vi "Scales Page.vi"() -> ()   [LabVIEW 2020, in "2D Plot.lvclass"]
uses:
  <vilib>/Math Plots/2D Math Plots/2D Plot/2D Plot/2D Plot.lvclass
  <vilib>/Math Plots/2D Math Plots/2D Plot/2D Plot/Typedef/Scale Array.ctl
  <vilib>/Math Plots/2D Math Plots/2D Plot/2D Plot/Typedef/Scale Cluster.ctl
  <vilib>/Utility/miscctls.llb/LVOffsetAndMultiplierTypeDef.ctl
  <vilib>/Math Plots/2D Math Plots/2D Plot/Action String/2DMathPlot Ctrl Act Queue.ctl
  <vilib>/Math Plots/2D Math Plots/2D Plot/Action String/2DMathPlot Ctrl Act Cluster.ctl
  <vilib>/Math Plots/2D Math Plots/2D Plot/Action String/2DMathPlot State Class.ctl
  <vilib>/Math Plots/2D Math Plots/2D Plot/2D Plot/Typedef/Dialog State.ctl
  <vilib>/Math Plots/2D Math Plots/2D Plot/2D Plot/Typedef/Temp Graph State.ctl
  <vilib>/Math Plots/2D Math Plots/2D Plot/2D Plot/Typedef/Temp Graph Property Action.ctl
panel:
  in  "Axis":string[](array[string])=["(X-Axis)", "(Y-Axis)"]
  in  "R Axis":string[](array[string])=["(R-Axis)"]
  in  "Event Registration":refnum<event-registration>
  in  "Control Ref Queue":T1
  out "Scale Array Out":T2
  in  "Scale Array In":T2
  in  "Current Scale":u16(ring) caption="Axes" items=["Time(X-Axis)", "Amplitude(Y-Axis)"]
  in  "Multiplier":dbl
  in  "Offset":dbl
  in  "Scale Style":u16(ring) caption="Scale Style and Colors"
  in  "Grid Style":u16(ring) caption="Grid Style and Colors"
  in  "Show Scale Label":bool caption="Show scale label"
  in  "Maximum":dbl=10.0
  in  "Minimum":dbl
  in  "Minor Grid":u32(colorbox)=13056 caption="Minor grid"
  in  "Major Grid":u32(colorbox)=26112 caption="Major grid"
  in  "Marker Text":u32(colorbox) caption="Marker text"
  in  "Minor Tick":u32(colorbox) caption="Minor tick"
  in  "Major Tick":u32(colorbox) caption="Major tick"
  in  "Autoscale":bool
  in  "Log":bool
  in  "Show Scale":bool caption="Show scale"
  in  "Inverted":bool
  in  "Name":string
  # "Scaling Factors"
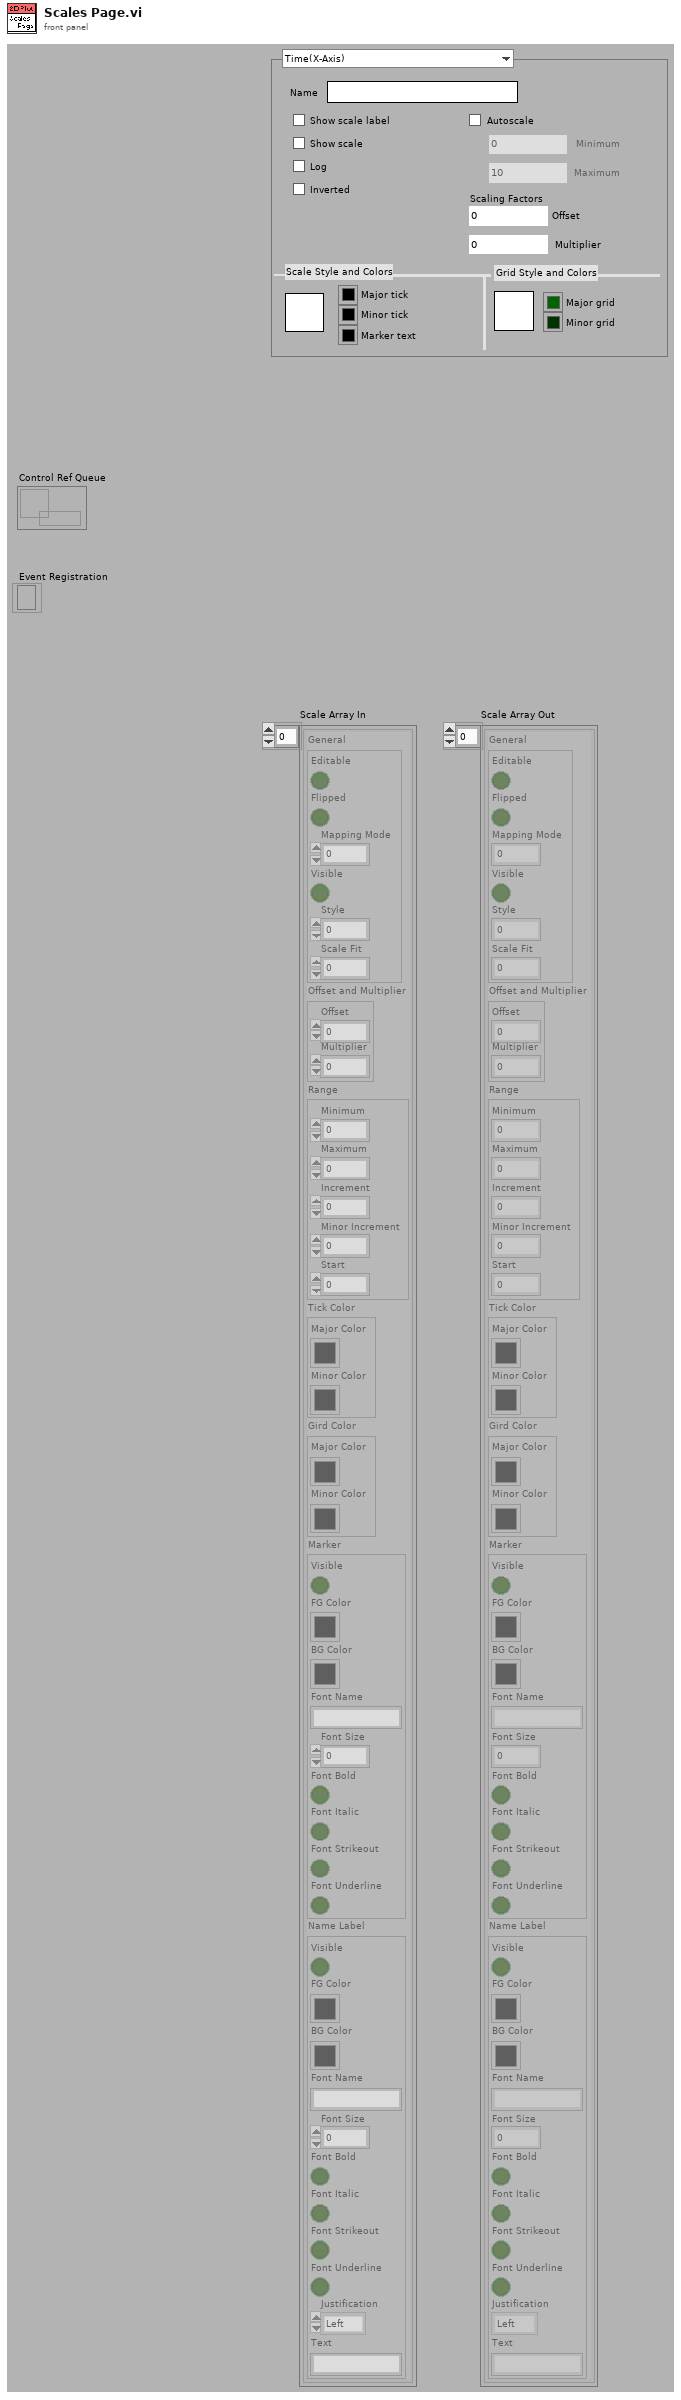
[diagram p1: front panel]
types:
  T1 = typedef "2DMathPlot Ctrl Act Queue.ctl" = refnum<queue>
  T2 = typedef "2D Plot.lvclass/Scale Array.ctl" = T3[]
  T3 = typedef "2D Plot.lvclass/Scale Cluster.ctl" = cluster{"General":cluster{"Editable":bool, "Flipped":bool, "Mapping Mode":u8, "Visible":bool, "Style":u8, "Scale Fit":u8}, "Offset and Multiplier":T4, "Range":cluster{"Minimum":dbl, "Maximum":dbl, "Increment":dbl, "Minor Increment":dbl, "Start":dbl}, "Tick Color":cluster{"Major Color":u32, "Minor Color":u32}, "Gird Color":cluster{"Major Color":u32, "Minor Color":u32}, "Marker":cluster{"Visible":bool, "FG Color":u32, "BG Color":u32, "Font Name":string, "Font Size":u32, "Font Bold":bool, "Font Italic":bool, "Font Strikeout":bool, "Font Underline":bool}, "Name Label":cluster{"Visible":bool, "FG Color":u32, "BG Color":u32, "Font Name":string, "Font Size":u32, "Font Bold":bool, "Font Italic":bool, "Font Strikeout":bool, "Font Underline":bool, "Justification":enum16{"Left", "Center", "Right"}, "Text":string}}
  T4 = typedef "LVOffsetAndMultiplierTypeDef.ctl" = cluster{"Offset":dbl, "Multiplier":dbl}
  T5 = typedef "2D Plot.lvclass/Dialog State.ctl" = enum16{"Initialize", "Read Property", "Write Property", "Idle", "Exit"}
  T6 = typedef "2DMathPlot Ctrl Act Cluster.ctl" = cluster{"Plot Area Ref":refnum<vi>, "Z Axis Ref":refnum<vi>, "Legend Ref":refnum<vi>, "XControl Ref":refnum<vi>, "Facade Ref":refnum<vi>, "Display State Change Class":T7}
  T7 = typedef "2DMathPlot State Class.ctl" = enum16{"Update All (Undo)", "Update General", "Update Appearance", "Update Format", "Update Scale", "Update Marker", "Update Cursor", "None"}
  T8 = typedef "2D Plot.lvclass/Temp Graph Property Action.ctl" = enum16{"Appearance Property", "Format Property", "Plots Property", "Scales Property"}
  T9 = typedef "2D Plot.lvclass/Temp Graph State.ctl" = enum16{"Create", "Update Graph", "Update Property Only", "Get Plot Name", "Get Axis Name", "Destory"}
  T10 = typedef "LVRangeTypeDef.ctl" = cluster{"Minimum":dbl, "Maximum":dbl, "Increment":dbl, "Minor Increment":dbl, "Start":dbl}
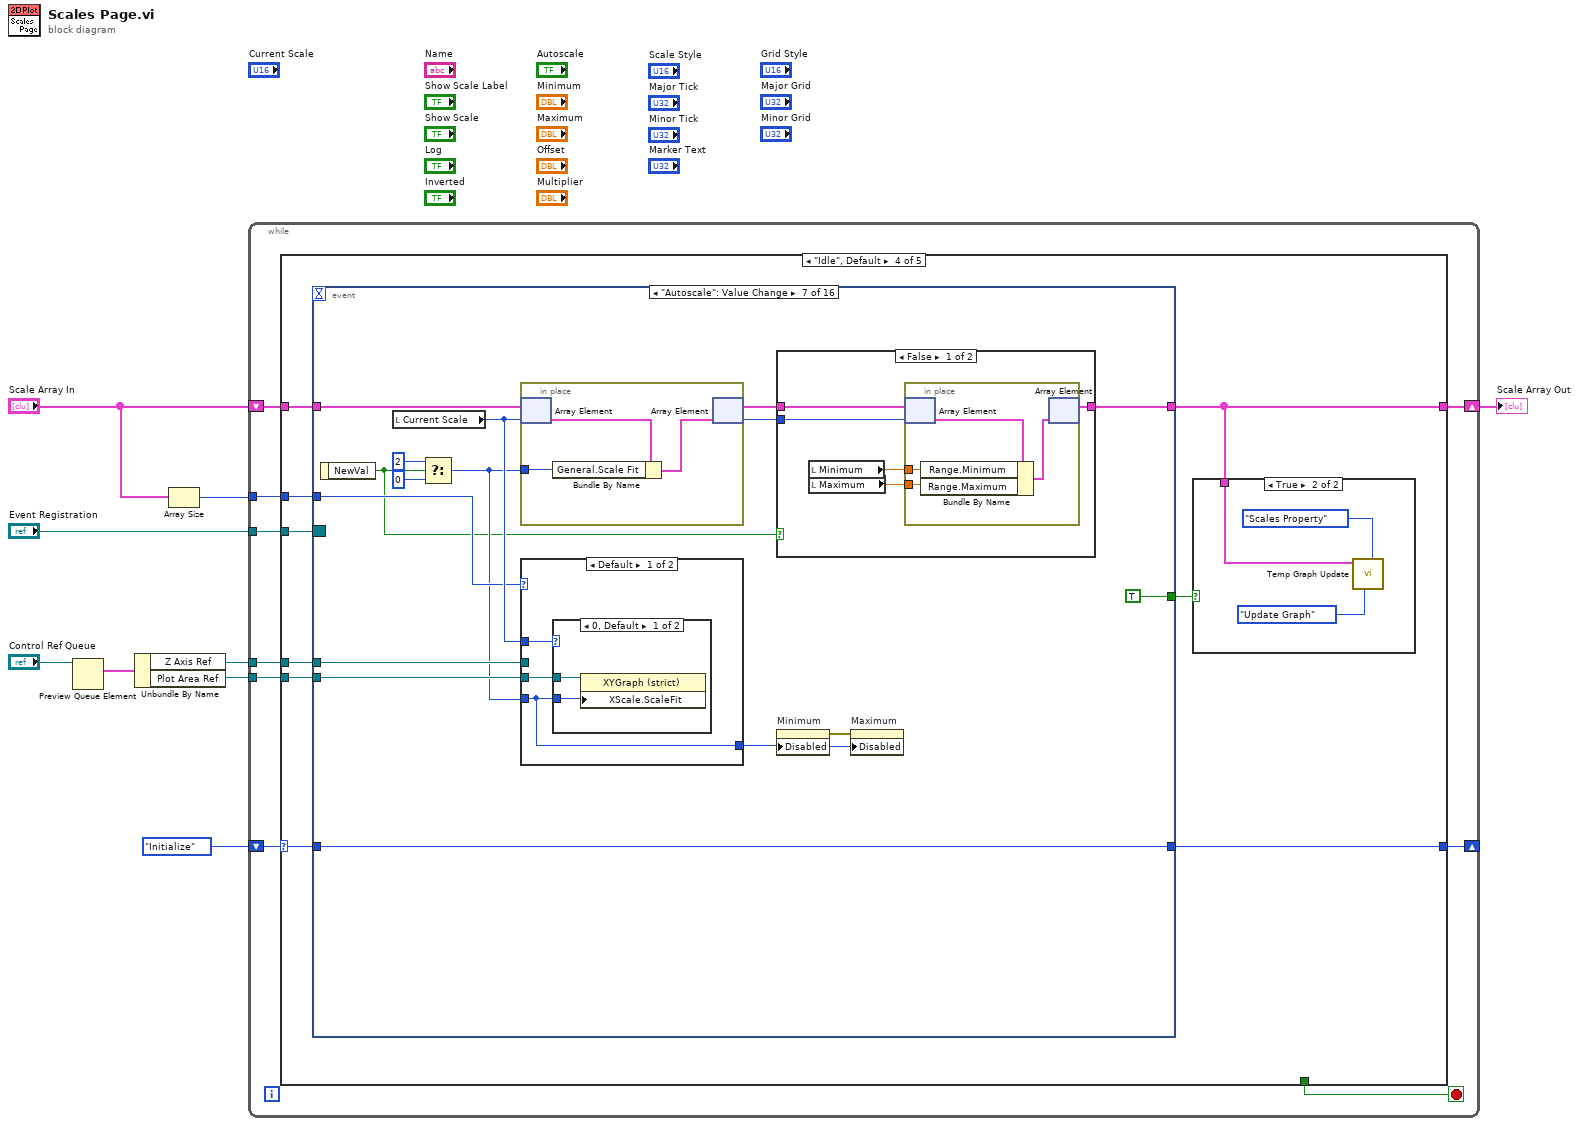
[diagram p0: block diagram]
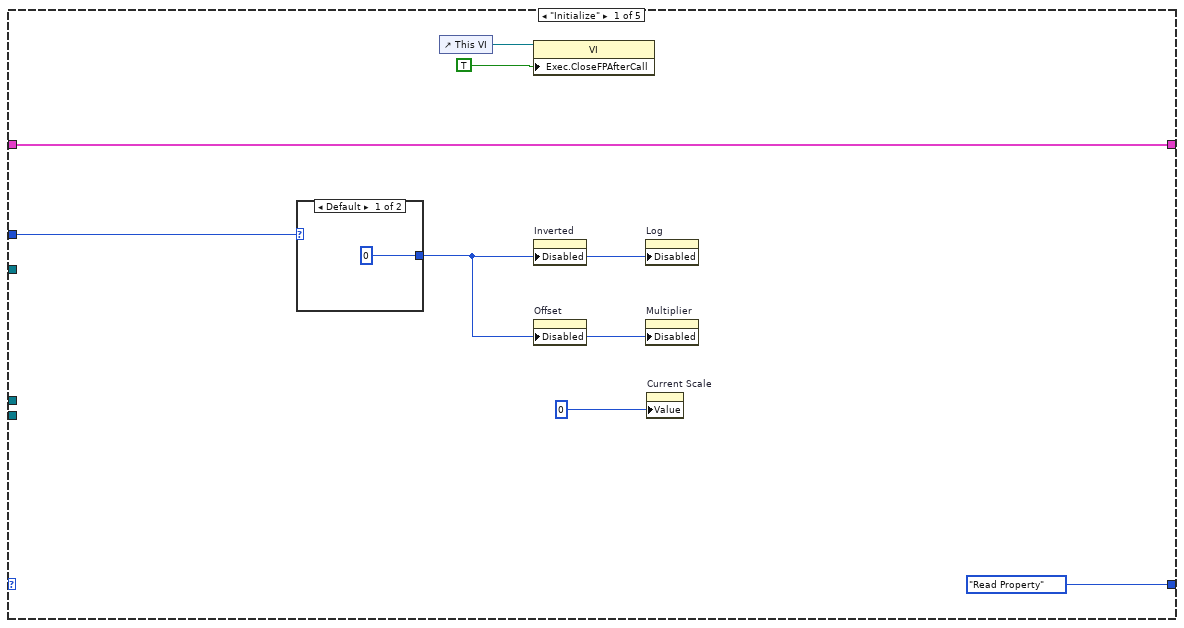
[diagram p2: hidden frame]
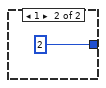
[diagram p3: hidden frame]
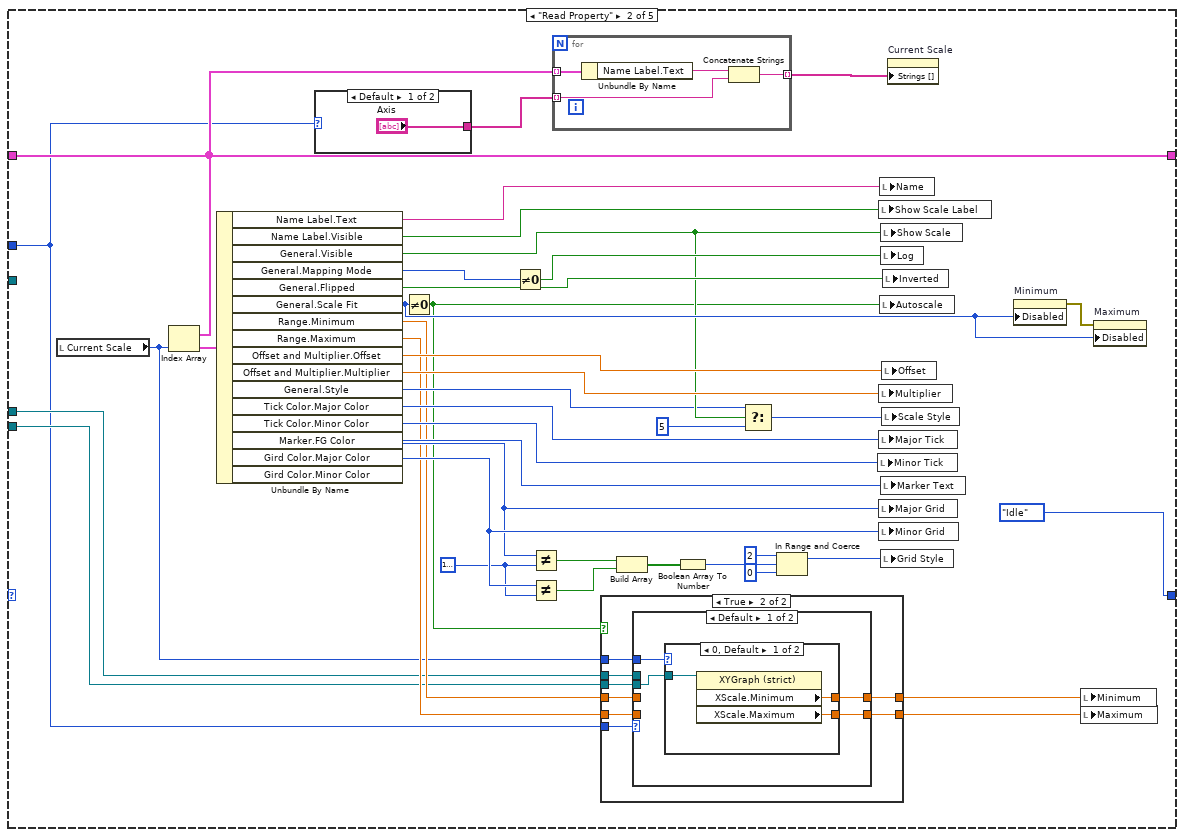
[diagram p4: hidden frame]
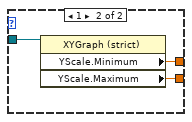
[diagram p6: hidden frame]
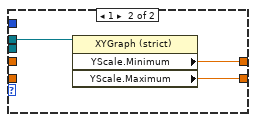
[diagram p7: hidden frame]
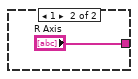
[diagram p8: hidden frame]
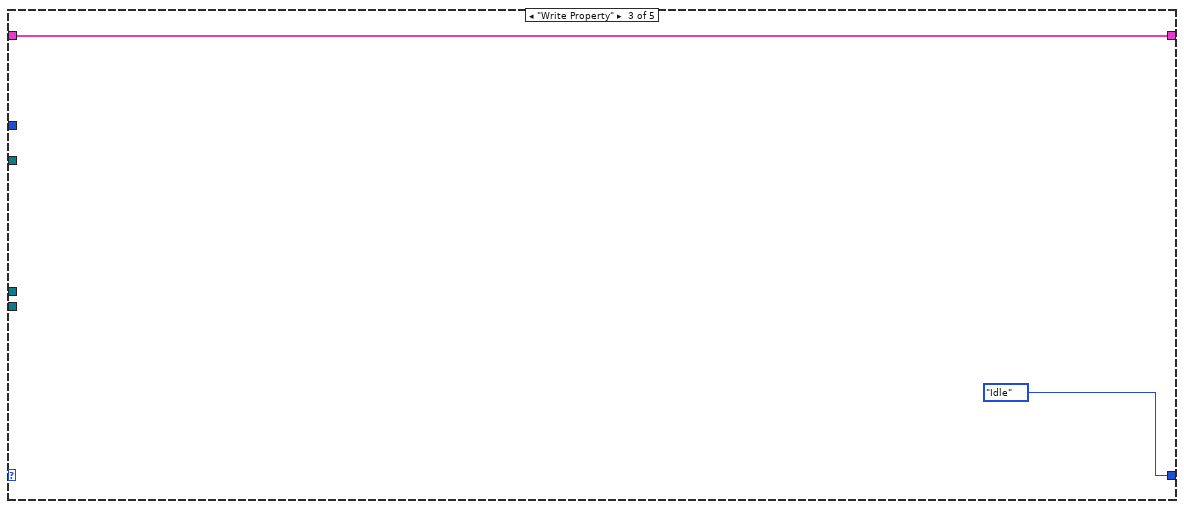
[diagram p9: hidden frame]
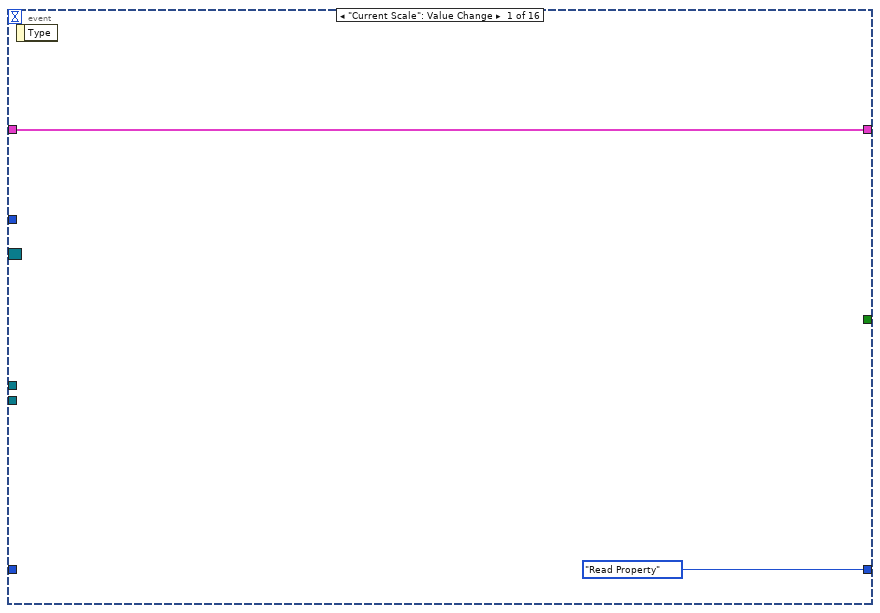
[diagram p11: hidden frame]
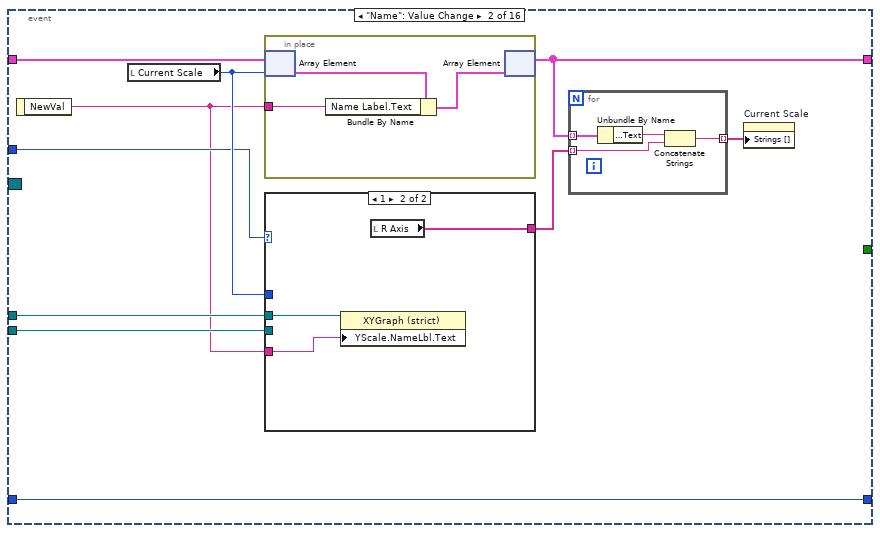
[diagram p12: hidden frame]
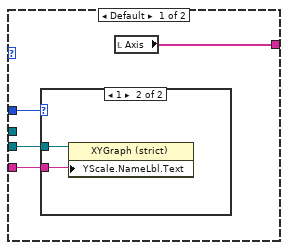
[diagram p13: hidden frame]
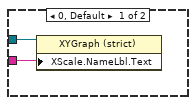
[diagram p14: hidden frame]
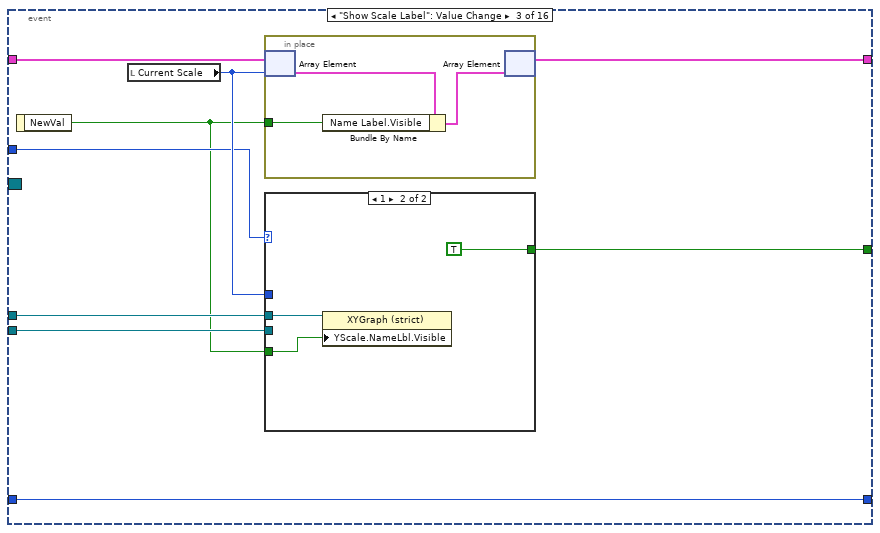
[diagram p15: hidden frame]
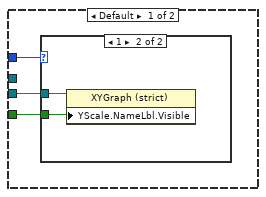
[diagram p16: hidden frame]
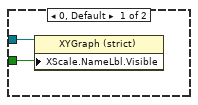
[diagram p17: hidden frame]
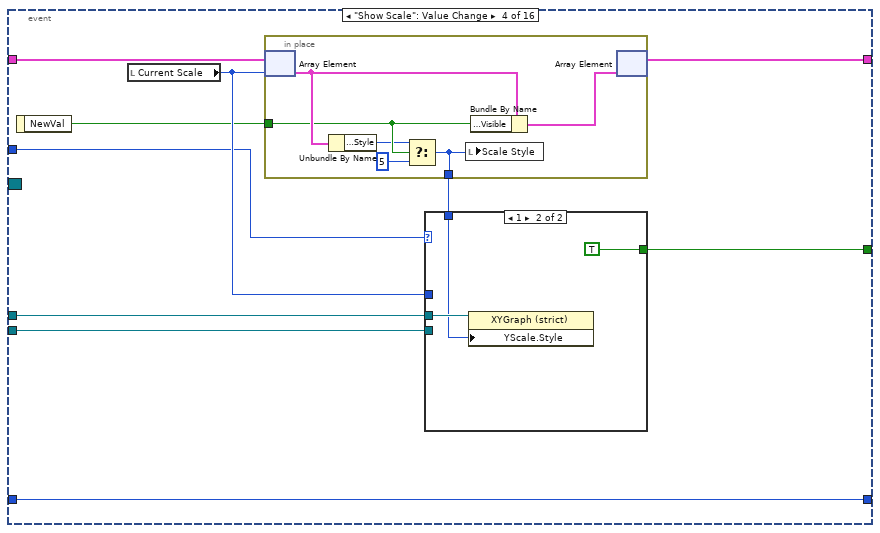
[diagram p18: hidden frame]
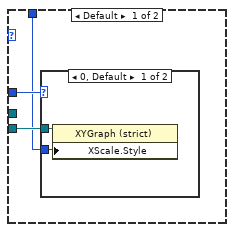
[diagram p19: hidden frame]
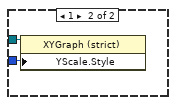
[diagram p20: hidden frame]
diagram:
  n1 = Preview Queue Element(queue="Control Ref Queue") -> (element=w6:T6)  [unwired: 1 in, 4 out]
  n2 = Unbundle By Name(w6) -> ("Z Axis Ref"=w4:refnum<vi>, "Plot Area Ref"=w3:refnum<vi>)
  n3 = Array Size(array="Scale Array In") -> (size(s)=w1:i32)
  n4 = while {
    shift-right: [w15] -> _
    shift-left: Dialog_State."Initialize" ("Enum") -> [w18]
    shift-right: [w16] -> w8
    shift-left: "Scale Array In" -> [w17]
    tunnel: "Event Registration" -> [w13]
    tunnel: w4 -> [w12]
    tunnel: w3 -> [w11]
    tunnel: w1 -> [w10]
    stop <- w14 stop-if-true
    n5 = case shown="\"Idle\", Default" w18 {
      selector: w18 -> [_ _ _ w102 w596]
      tunnel: w17 -> [w23 w37 w98 w107 w594]
      tunnel: [w23 w37 w98 w101 w594] -> w16
      tunnel: [Dialog_State."Read Property" ("Enum") Dialog_State."Idle" ("Enum") Dialog_State."Idle" ("Enum") w100 w596] -> w15
      tunnel: [_ _ _ _ TRUE] -> w14
      tunnel: w13 -> [_ _ _ w106 _]
      tunnel: w12 -> [_ w32 _ w105 _]
      tunnel: w11 -> [_ w30 _ w104 _]
      tunnel: w10 -> [w21 w29 _ w103 _]
      frame "Initialize" {
        n6 = case shown="Default" w21 {
          tunnel: [u8 0 ("Disabled") u8 2 ("Disabled")] -> w20
          frame Default {
          }
          frame 1 {
          }
        }
        n7 = control-ref of="This VI"() -> (w25:refnum<vi>)
        n8 = property class="VI"(reference=w25, "Exec.CloseFPAfterCall"=TRUE ("Execution:Close After Call")) -> ()  [unwired: 1 in, 2 out]
        n9 = property on="Inverted" class="Bool (strict)"("Disabled"=w20) -> ()  [unwired: 2 in, 2 out]
        n10 = property on="Offset" class="DigNum (strict)"("Disabled"=w20) -> ()  [unwired: 2 in, 2 out]
        n11 = property on="Log" class="Bool (strict)"("Disabled"=w20) -> ()  [unwired: 2 in, 2 out]
        n12 = property on="Multiplier" class="DigNum (strict)"("Disabled"=w20) -> ()  [unwired: 2 in, 2 out]
        n13 = property on="Current Scale" class="Ring (strict)"("Value"=u16 0) -> ()  [unwired: 2 in, 2 out]
      }
      frame "Read Property" {
        w48 = u32 16777216
        n14 = local read "Current Scale"() -> (w31:u16)
        n15 = Index Array(array=w37, index=w31) -> (element=w67:T3)
        n16 = Unbundle By Name(w67) -> ("Name Label.Text"=w66:string, "Name Label.Visible"=w65:bool, "General.Visible"=w41:bool, "General.Mapping Mode"=w64:u8, "General.Flipped"=w62:bool, "General.Scale Fit"=w61:u8, "Range.Minimum"=w36:dbl, "Range.Maximum"=w34:dbl, "Offset and Multiplier.Offset"=w59:dbl, "Offset and Multiplier.Multiplier"=w58:dbl, "General.Style"=w40:u8, "Tick Color.Major Color"=w57:u32, "Tick Color.Minor Color"=w55:u32, "Marker.FG Color"=w56:u32, "Gird Color.Major Color"=w52:u32, "Gird Color.Minor Color"=w53:u32)
        n17 = case shown="Default" w29 {
          tunnel: ["Axis" "R Axis"] -> w46
          frame Default {
          }
          frame 1 {
          }
        }
        n18 = Not Equal To 0?(x=w61) -> (x != 0?=w28:bool)
        n19 = Not Equal To 0?(x=w64) -> (x != 0?=w63:bool)
        n20 = Not Equal?(x=w52, y=w48) -> (x != y?=w50:bool)
        n21 = Not Equal?(x=w53, y=w48) -> (x != y?=w51:bool)
        n22 = for {
          tunnel: w37 -> [w96] mode=indexing
          tunnel: w46 -> [w94] mode=indexing
          tunnel: [w93] -> w47 mode=indexing
          n23 = Unbundle By Name(w96) -> ("Name Label.Text"=w95:string)
          n24 = Concatenate Strings(w95, w94) -> (w93:string)
        }
        n25 = case shown="True" w28 {
          tunnel: w36 -> [w69 w77]
          tunnel: [w69 w76] -> w35
          tunnel: w34 -> [w68 w75]
          tunnel: [w68 w74] -> w33
          tunnel: w32 -> [_ w73]
          tunnel: w31 -> [_ w72]
          tunnel: w30 -> [_ w71]
          tunnel: w29 -> [_ w70]
          frame False {
          }
          frame True {
            n26 = case shown="Default" w70 {
              tunnel: w77 -> [_ _]
              tunnel: [w79 w90] -> w76
              tunnel: w75 -> [_ _]
              tunnel: [w78 w89] -> w74
              tunnel: w73 -> [_ w88]
              tunnel: w72 -> [w81 _]
              tunnel: w71 -> [w80 _]
              frame Default {
                n27 = case shown="0, Default" w81 {
                  tunnel: w80 -> [w84 w87]
                  tunnel: [w83 w86] -> w79
                  tunnel: [w82 w85] -> w78
                  frame 0, Default {
                    n28 = property class="XYGraph (strict)"(reference=w84) -> ("XScale.Minimum"=w83:dbl, "XScale.Maximum"=w82:dbl)  [unwired: 1 in, 2 out]
                  }
                  frame 1 {
                    n29 = property class="XYGraph (strict)"(reference=w87) -> ("YScale.Minimum"=w86:dbl, "YScale.Maximum"=w85:dbl)  [unwired: 1 in, 2 out]
                  }
                }
              }
              frame 1 {
                n30 = property class="XYGraph (strict)"(reference=w88) -> ("YScale.Minimum"=w90:dbl, "YScale.Maximum"=w89:dbl)  [unwired: 1 in, 2 out]
              }
            }
          }
        }
        n31 = Build Array(w50, w51) -> (w49:bool[])
        n32 = Boolean Array To Number(Boolean array=w49) -> (number=w45:u16)
        n33 = Select(t=w40, s=w41, f=u8 5) -> (s? t:f=w38:u8)
        n34 = In Range and Coerce(upper limit=u16 2, x=w45, lower limit=u16 0) -> (coerced(x)=w42:u16)  [unwired: 1 out]
        n35 = local write "Minor Tick"(w55) -> ()
        n36 = local write "Show Scale Label"(w65) -> ()
        n37 = local write "Multiplier"(w58) -> ()
        n38 = local write "Major Tick"(w57) -> ()
        n39 = local write "Major Grid"(w52) -> ()
        n40 = local write "Minor Grid"(w53) -> ()
        n41 = local write "Name"(w66) -> ()
        n42 = local write "Autoscale"(w28) -> ()
        n43 = local write "Show Scale"(w41) -> ()
        n44 = local write "Log"(w63) -> ()
        n45 = local write "Marker Text"(w56) -> ()
        n46 = local write "Grid Style"(w42) -> ()
        n47 = local write "Offset"(w59) -> ()
        n48 = local write "Scale Style"(w38) -> ()
        n49 = local write "Inverted"(w62) -> ()
        n50 = property on="Current Scale" class="Ring (strict)"("Strings []"=w47) -> ()  [unwired: 2 in, 2 out]
        n51 = property on="Minimum" class="DigNum (strict)"("Disabled"=w61) -> (error out=w54:errorcluster)  [unwired: 2 in, 1 out]
        n52 = local write "Minimum"(w35) -> ()
        n53 = local write "Maximum"(w33) -> ()
        n54 = property on="Maximum" class="DigNum (strict)"(error in=w54, "Disabled"=w61) -> ()  [unwired: 1 in, 2 out]
      }
      frame "Write Property" {
      }
      frame "Idle", Default {
        n55 = event shown="[6] \"Autoscale\": Value Change" {
          selector: w106 -> [_ _ _ _ _ _ _ _ _ _ _ _ _ _ _ _]
          dyn-events: _ -> [_ _ _ _ _ _ _ _ _ _ _ _ _ _ _ _]
          timeout: _ -> [_ _ _ _ _ _ _ _ _ _ _ _ _ _ _ _]
          tunnel: w107 -> [w112 w122 w149 w172 w200 w218 w244 w272 w338 w365 w414 w436 w461 w481 w576 w593]
          tunnel: [w112 w120 w148 w171 w199 w217 w231 w271 w337 w364 w413 w435 w460 w480 w575 w593] -> w101
          tunnel: [Dialog_State."Read Property" ("Enum") w113 w142 w165 w194 w212 w237 w273 w336 w363 w407 w428 w454 w475 w564 Dialog_State."Exit" ("Enum")] -> w100
          tunnel: w105 -> [_ w115 w144 w167 w195 _ w240 w274 _ _ w409 w431 w456 w477 w571 _]
          tunnel: w104 -> [_ w119 w147 w170 w198 w216 w243 w276 w334 w362 w412 w434 w459 w479 w574 _]
          tunnel: w103 -> [_ w117 w145 w168 w196 w214 w241 w275 w330 w361 w410 w432 w457 w478 w572 _]
          tunnel: w102 -> [_ w113 w142 w165 w194 w212 w237 w273 w336 w363 w407 w428 w454 w475 w564 _]
          tunnel: [_ _ w141 w163 TRUE TRUE TRUE w267 TRUE w359 w406 _ _ w474 w559 _] -> w99
          event "Current Scale": Value Change {
            n56 = event-data() -> ()  [unwired: 2 out]
          }
          event "Name": Value Change {
            n57 = event-data() -> ("NewVal"=w114:string)  [unwired: 1 out]
            n58 = local read "Current Scale"() -> (w118:u16)
            n59 = in-place {
              in-place-border: w114 -> [w138]
              n60 = in-place-array #1(w122, w118) -> (w140:T3)
              n61 = Bundle By Name(cluster=w140, "Name Label.Text"=w138) -> (w139:T3)
              n62 = in-place-array #1(w139) -> (w120:T2)  [unwired: 1 out]
            }
            n63 = case shown="1" w117 {
              tunnel: [w123 w131] -> w116
              tunnel: w119 -> [w126 _]
              tunnel: w118 -> [w125 _]
              tunnel: w115 -> [_ w133]
              tunnel: w114 -> [w124 w132]
              frame Default {
                n64 = case shown="1" w125 {
                  tunnel: w126 -> [w128 w130]
                  tunnel: w124 -> [w127 w129]
                  frame 0, Default {
                    n65 = property class="XYGraph (strict)"(reference=w128, "XScale.NameLbl.Text"=w127) -> ()  [unwired: 1 in, 2 out]
                  }
                  frame 1 {
                    n66 = property class="XYGraph (strict)"(reference=w130, "YScale.NameLbl.Text"=w129) -> ()  [unwired: 1 in, 2 out]
                  }
                }
                n67 = local read "Axis"() -> (w123:string[])
              }
              frame 1 {
                n68 = property class="XYGraph (strict)"(reference=w133, "YScale.NameLbl.Text"=w132) -> ()  [unwired: 1 in, 2 out]
                n69 = local read "R Axis"() -> (w131:string[])
              }
            }
            n70 = for {
              tunnel: w120 -> [w137] mode=indexing
              tunnel: w116 -> [w135] mode=indexing
              tunnel: [w134] -> w121 mode=indexing
              n71 = Unbundle By Name(w137) -> ("Name Label.Text"=w136:string)
              n72 = Concatenate Strings(w136, w135) -> (w134:string)
            }
            n73 = property on="Current Scale" class="Ring (strict)"("Strings []"=w121) -> ()  [unwired: 2 in, 2 out]
          }
          event "Show Scale Label": Value Change {
            n74 = event-data() -> ("NewVal"=w143:bool)  [unwired: 1 out]
            n75 = local read "Current Scale"() -> (w146:u16)
            n76 = in-place {
              in-place-border: w143 -> [w160]
              n77 = in-place-array #2(w149, w146) -> (w162:T3)
              n78 = Bundle By Name(cluster=w162, "Name Label.Visible"=w160) -> (w161:T3)
              n79 = in-place-array #2(w161) -> (w148:T2)  [unwired: 1 out]
            }
            n80 = case shown="1" w145 {
              tunnel: w147 -> [w152 _]
              tunnel: w146 -> [w151 _]
              tunnel: w144 -> [_ w158]
              tunnel: w143 -> [w150 w157]
              tunnel: [_ TRUE] -> w141
              frame Default {
                n81 = case shown="1" w151 {
                  tunnel: w152 -> [w154 w156]
                  tunnel: w150 -> [w153 w155]
                  frame 0, Default {
                    n82 = property class="XYGraph (strict)"(reference=w154, "XScale.NameLbl.Visible"=w153) -> ()  [unwired: 1 in, 2 out]
                  }
                  frame 1 {
                    n83 = property class="XYGraph (strict)"(reference=w156, "YScale.NameLbl.Visible"=w155) -> ()  [unwired: 1 in, 2 out]
                  }
                }
              }
              frame 1 {
                n84 = property class="XYGraph (strict)"(reference=w158, "YScale.NameLbl.Visible"=w157) -> ()  [unwired: 1 in, 2 out]
              }
            }
          }
          event "Show Scale": Value Change {
            n85 = event-data() -> ("NewVal"=w166:bool)  [unwired: 1 out]
            n86 = local read "Current Scale"() -> (w169:u16)
            n87 = in-place {
              in-place-border: w166 -> [w185]
              in-place-border: [w183] -> w164
              n88 = in-place-array #3(w172, w169) -> (w187:T3)
              n89 = Unbundle By Name(w187) -> ("General.Style"=w184:u8)
              n90 = Select(t=w184, s=w185, f=u8 5) -> (s? t:f=w183:u8)
              n91 = local write "Scale Style"(w183) -> ()
              n92 = Bundle By Name(cluster=w187, "General.Visible"=w185) -> (w188:T3)
              n93 = in-place-array #3(w188) -> (w171:T2)  [unwired: 1 out]
            }
            n94 = case shown="1" w168 {
              tunnel: w170 -> [w175 _]
              tunnel: w169 -> [w174 _]
              tunnel: w167 -> [_ w182]
              tunnel: w164 -> [w173 w181]
              tunnel: [_ TRUE] -> w163
              frame Default {
                n95 = case shown="0, Default" w174 {
                  tunnel: w175 -> [w177 w179]
                  tunnel: w173 -> [w176 w178]
                  frame 0, Default {
                    n96 = property class="XYGraph (strict)"(reference=w177, "XScale.Style"=w176) -> ()  [unwired: 1 in, 2 out]
                  }
                  frame 1 {
                    n97 = property class="XYGraph (strict)"(reference=w179, "YScale.Style"=w178) -> ()  [unwired: 1 in, 2 out]
                  }
                }
              }
              frame 1 {
                n98 = property class="XYGraph (strict)"(reference=w182, "YScale.Style"=w181) -> ()  [unwired: 1 in, 2 out]
              }
            }
          }
          event "Log": Value Change {
            w191 = u8 0 ("General.Mapping Mode")
            n99 = event-data() -> ("NewVal"=w193:bool)  [unwired: 1 out]
            n100 = Increment(x=w191) -> (x+1=w190:u8)
            n101 = local read "Current Scale"() -> (w197:u16)
            n102 = Select(t=w190, s=w193, f=w191) -> (s? t:f=w192:u8)
            n103 = in-place {
              in-place-border: w192 -> [w208]
              n104 = in-place-array #4(w200, w197) -> (w210:T3)
              n105 = Bundle By Name(cluster=w210, "General.Mapping Mode"=w208) -> (w209:T3)
              n106 = in-place-array #4(w209) -> (w199:T2)  [unwired: 1 out]
            }
            n107 = case shown="Default" w196 {
              tunnel: w198 -> [w203 _]
              tunnel: w197 -> [w202 _]
              tunnel: w195 -> [_ _]
              tunnel: w192 -> [w201 _]
              frame Default {
                n108 = case shown="0, Default" w202 {
                  tunnel: w203 -> [w205 w207]
                  tunnel: w201 -> [w204 w206]
                  frame 0, Default {
                    n109 = property class="XYGraph (strict)"(reference=w205, "XScale.Mapping Mode"=w204) -> ()  [unwired: 1 in, 2 out]
                  }
                  frame 1 {
                    n110 = property class="XYGraph (strict)"(reference=w207, "YScale.Mapping Mode"=w206) -> ()  [unwired: 1 in, 2 out]
                  }
                }
              }
              frame 1 {
                # "Compass plot do not have log scale."
              }
            }
          }
          event "Inverted": Value Change {
            n111 = event-data() -> ("NewVal"=w213:bool)  [unwired: 1 out]
            n112 = local read "Current Scale"() -> (w215:u16)
            n113 = in-place {
              in-place-border: w213 -> [w226]
              n114 = in-place-array #5(w218, w215) -> (w228:T3)
              n115 = Bundle By Name(cluster=w228, "General.Flipped"=w226) -> (w227:T3)
              n116 = in-place-array #5(w227) -> (w217:T2)  [unwired: 1 out]
            }
            n117 = case shown="Default" w214 {
              tunnel: w216 -> [w221 _]
              tunnel: w215 -> [w220 _]
              tunnel: w213 -> [w219 _]
              frame Default {
                n118 = case shown="0, Default" w220 {
                  tunnel: w221 -> [w223 w225]
                  tunnel: w219 -> [w222 w224]
                  frame 0, Default {
                    n119 = property class="XYGraph (strict)"(reference=w223, "XScale.Flipped"=w222) -> ()  [unwired: 1 in, 2 out]
                  }
                  frame 1 {
                    n120 = property class="XYGraph (strict)"(reference=w225, "YScale.Flipped"=w224) -> ()  [unwired: 1 in, 2 out]
                  }
                }
              }
              frame 1 {
                # "Compass plot do no have flip scale."
              }
            }
          }
          event "Autoscale": Value Change {
            n121 = event-data() -> ("NewVal"=w229:bool)  [unwired: 1 out]
            n122 = local read "Current Scale"() -> (w242:u16)
            n123 = Select(t=u8 2 ("General.Scale Fit"), s=w229, f=u8 0) -> (s? t:f=w236:u8)
            n124 = in-place {
              in-place-border: w236 -> [w264]
              n125 = in-place-array #6(w244, w242) -> (w266:T3)
              n126 = Bundle By Name(cluster=w266, "General.Scale Fit"=w264) -> (w265:T3)
              n127 = in-place-array #6(w265) -> (w232:T2, w230:i32)
            }
            n128 = case shown="Default" w241 {
              tunnel: w243 -> [w257 _]
              tunnel: w242 -> [w256 _]
              tunnel: w240 -> [_ w263]
              tunnel: w236 -> [w255 w262]
              tunnel: [w255 w262] -> w238
              frame Default {
                n129 = case shown="0, Default" w256 {
                  tunnel: w257 -> [w259 w261]
                  tunnel: w255 -> [w258 w260]
                  frame 0, Default {
                    n130 = property class="XYGraph (strict)"(reference=w259, "XScale.ScaleFit"=w258) -> ()  [unwired: 1 in, 2 out]
                  }
                  frame 1 {
                    n131 = property class="XYGraph (strict)"(reference=w261, "YScale.ScaleFit"=w260) -> ()  [unwired: 1 in, 2 out]
                  }
                }
              }
              frame 1 {
                n132 = property class="XYGraph (strict)"(reference=w263, "YScale.ScaleFit"=w262) -> ()  [unwired: 1 in, 2 out]
              }
            }
            n133 = case shown="False" w229 {
              tunnel: w232 -> [w249 w254]
              tunnel: [w248 w254] -> w231
              tunnel: w230 -> [w245 _]
              frame False {
                n134 = local read "Minimum"() -> (w247:dbl)
                n135 = local read "Maximum"() -> (w246:dbl)
                n136 = in-place {
                  in-place-border: w247 -> [w251]
                  in-place-border: w246 -> [w250]
                  n137 = in-place-array #7(w249, w245) -> (w253:T3)
                  n138 = Bundle By Name(cluster=w253, "Range.Minimum"=w251, "Range.Maximum"=w250) -> (w252:T3)
                  n139 = in-place-array #7(w252) -> (w248:T2)  [unwired: 1 out]
                }
              }
              frame True {
              }
            }
            n140 = property on="Minimum" class="DigNum (strict)"("Disabled"=w238) -> (error out=w239:errorcluster)  [unwired: 2 in, 1 out]
            n141 = property on="Maximum" class="DigNum (strict)"(error in=w239, "Disabled"=w238) -> ()  [unwired: 1 in, 2 out]
          }
          event "Minimum", "Maximum": Value Change {
            n142 = event-data() -> ()  [unwired: 2 out]
            n143 = local read "Current Scale"() -> (w270:u16)
            n144 = local read "Minimum"() -> (w269:dbl)
            n145 = local read "Maximum"() -> (w268:dbl)
            n146 = case shown="1" w275 {
              tunnel: w276 -> [w283 _]
              tunnel: w274 -> [_ w303]
              tunnel: w272 -> [w282 w300]
              tunnel: [w281 w298] -> w271
              tunnel: w270 -> [w278 w299]
              tunnel: w269 -> [w280 w297]
              tunnel: w268 -> [w279 w296]
              tunnel: [TRUE w294] -> w267
              frame Default {
                n147 = in-place {
                  in-place-border: w280 -> [w285]
                  in-place-border: w279 -> [w284]
                  n148 = in-place-array #8(w282, w278) -> (w287:T3)
                  n149 = Bundle By Name(cluster=w287, "Range.Minimum"=w285, "Range.Maximum"=w284) -> (w286:T3)
                  n150 = in-place-array #8(w286) -> (w281:T2)  [unwired: 1 out]
                }
                n151 = case shown="0, Default" w278 {
                  tunnel: w283 -> [w290 w292]
                  tunnel: w280 -> [w289 w293]
                  tunnel: w279 -> [w288 w291]
                  frame 0, Default {
                    n152 = property class="XYGraph (strict)"(reference=w290, "XScale.Minimum"=w289, "XScale.Maximum"=w288) -> ()  [unwired: 1 in, 2 out]
                  }
                  frame 1 {
                    n153 = property class="XYGraph (strict)"(reference=w292, "YScale.Minimum"=w293, "YScale.Maximum"=w291) -> ()  [unwired: 1 in, 2 out]
                  }
                }
              }
              frame 1 {
                n154 = Less Than 0?(x=w297) -> (x < 0?=w301:bool)
                n155 = Less Than 0?(x=w296) -> (x < 0?=w302:bool)
                n156 = Or(x=w301, y=w302) -> (x .or. y?=w295:bool)
                n157 = case shown="False" w295 {
                  tunnel: w303 -> [w312 _]
                  tunnel: w297 -> [w311 _]
                  tunnel: w296 -> [w310 _]
                  tunnel: w300 -> [w309 w321]
                  tunnel: w299 -> [w308 w318]
                  tunnel: [w307 w321] -> w298
                  tunnel: w297 -> [w306 _]
                  tunnel: w296 -> [w305 _]
                  tunnel: [TRUE FALSE] -> w294
                  frame False {
                    n158 = in-place {
                      in-place-border: w306 -> [w314]
                      in-place-border: w305 -> [w313]
                      n159 = in-place-array #9(w309, w308) -> (w316:T3)
                      n160 = Bundle By Name(cluster=w316, "Range.Minimum"=w314, "Range.Maximum"=w313) -> (w315:T3)
                      n161 = in-place-array #9(w315) -> (w307:T2)  [unwired: 1 out]
                    }
                    n162 = property class="XYGraph (strict)"(reference=w312, "YScale.Minimum"=w311, "YScale.Maximum"=w310) -> ()  [unwired: 1 in, 2 out]
                  }
                  frame True {
                    n163 = Index Array(array=w321, index=w318) -> (element=w322:T3)
                    n164 = Unbundle By Name(w322) -> ("Range.Minimum"=w319:dbl, "Range.Maximum"=w320:dbl)
                    n165 = local write "Minimum"(w319) -> ()
                    n166 = local write "Maximum"(w320) -> ()
                  }
                }
              }
            }
          }
          event "Offset": Value Change {
            n167 = event-data() -> ("NewVal"=w329:dbl, "OldVal"=w326:dbl)  [unwired: 1 out]
            n168 = local read "Current Scale"() -> (w335:u16)
            n169 = local read "Minimum"() -> (w328:dbl)
            n170 = local read "Maximum"() -> (w327:dbl)
            n171 = Subtract(x=w328, y=w326) -> (x-y=w325:dbl)
            n172 = Subtract(x=w327, y=w326) -> (x-y=w324:dbl)
            n173 = Add(x=w329, y=w325) -> (x+y=w333:dbl)
            n174 = Add(x=w329, y=w324) -> (x+y=w332:dbl)
            n175 = case shown="0, Default" w335 {
              tunnel: w334 -> [w342 w345]
              tunnel: w333 -> [w341 w346]
              tunnel: w332 -> [w340 w344]
              tunnel: [w339 w343] -> w331
              frame 0, Default {
                n176 = property class="XYGraph (strict)"(reference=w342, "XScale.Minimum"=w341, "XScale.Maximum"=w340) -> ("XScale.Range"=w339:T10)  [unwired: 1 in, 2 out]
              }
              frame 1 {
                n177 = property class="XYGraph (strict)"(reference=w345, "YScale.Minimum"=w346, "YScale.Maximum"=w344) -> ("YScale.Range"=w343:T10)  [unwired: 1 in, 2 out]
              }
            }
            n178 = in-place {
              in-place-border: w329 -> [w351]
              in-place-border: w331 -> [w347]
              in-place-border: w330 -> [w348]
              n179 = in-place-array #10(w338, w335) -> (w352:T3)
              n180 = Bundle By Name(cluster=w352, "Offset and Multiplier.Offset"=w351) -> (w350:T3)
              n181 = case shown="Default" w348 {
                tunnel: w350 -> [w353 w356]
                tunnel: [w353 w355] -> w349
                tunnel: w347 -> [_ w354]
                frame 1 {
                }
                frame Default {
                  n182 = Bundle By Name(cluster=w356, "Range"=w354) -> (w355:T3)
                }
              }
              n183 = in-place-array #10(w349) -> (w337:T2)  [unwired: 1 out]
            }
            n184 = local write "Minimum"(w333) -> ()
            n185 = local write "Maximum"(w332) -> ()
          }
          event "Multiplier": Value Change {
            n186 = event-data() -> ("NewVal"=w358:dbl, "OldVal"=w360:dbl)  [unwired: 1 out]
            n187 = Not Equal To 0?(x=w358) -> (x != 0?=w357:bool)
            n188 = case shown="True" w357 {
              tunnel: w365 -> [w367 w387]
              tunnel: [w367 w386] -> w364
              tunnel: w362 -> [_ w382]
              tunnel: w361 -> [_ w378]
              tunnel: w358 -> [_ w377]
              tunnel: w360 -> [w366 w372]
              tunnel: [_ TRUE] -> w359
              frame False {
                n189 = local write "Multiplier"(w366) -> ()
              }
              frame True {
                n190 = local read "Minimum"() -> (w376:dbl)
                n191 = local read "Maximum"() -> (w375:dbl)
                n192 = local read "Offset"() -> (w369:dbl)
                n193 = Subtract(x=w376, y=w369) -> (x-y=w373:dbl)
                n194 = Subtract(x=w375, y=w369) -> (x-y=w374:dbl)
                n195 = local read "Current Scale"() -> (w383:u16)
                n196 = Divide(x=w373, y=w372) -> (x/y=w371:dbl)
                n197 = Divide(x=w374, y=w372) -> (x/y=w370:dbl)
                n198 = Multiply(x=w377, y=w371) -> (x*y=w385:dbl)
                n199 = Multiply(x=w377, y=w370) -> (x*y=w384:dbl)
                n200 = Add(x=w369, y=w385) -> (x+y=w381:dbl)
                n201 = Add(x=w369, y=w384) -> (x+y=w380:dbl)
                n202 = case shown="1" w383 {
                  tunnel: w382 -> [w391 w394]
                  tunnel: w381 -> [w390 w395]
                  tunnel: w380 -> [w389 w393]
                  tunnel: [w388 w392] -> w379
                  frame 0, Default {
                    n203 = property class="XYGraph (strict)"(reference=w391, "XScale.Minimum"=w390, "XScale.Maximum"=w389) -> ("XScale.Range"=w388:T10)  [unwired: 1 in, 2 out]
                  }
                  frame 1 {
                    n204 = property class="XYGraph (strict)"(reference=w394, "YScale.Minimum"=w395, "YScale.Maximum"=w393) -> ("YScale.Range"=w392:T10)  [unwired: 1 in, 2 out]
                  }
                }
                n205 = in-place {
                  in-place-border: w377 -> [w400]
                  in-place-border: w379 -> [w396]
                  in-place-border: w378 -> [w397]
                  n206 = in-place-array #11(w387, w383) -> (w401:T3)
                  n207 = Bundle By Name(cluster=w401, "Offset and Multiplier.Multiplier"=w400) -> (w399:T3)
                  n208 = case shown="Default" w397 {
                    tunnel: w399 -> [w402 w405]
                    tunnel: [w402 w404] -> w398
                    tunnel: w396 -> [_ w403]
                    frame 1 {
                    }
                    frame Default {
                      n209 = Bundle By Name(cluster=w405, "Range"=w403) -> (w404:T3)
                    }
                  }
                  n210 = in-place-array #11(w398) -> (w386:T2)  [unwired: 1 out]
                }
                n211 = local write "Minimum"(w381) -> ()
                n212 = local write "Maximum"(w380) -> ()
              }
            }
          }
          event "Scale Style": Value Change {
            n213 = event-data() -> ("NewVal"=w408:u16)  [unwired: 1 out]
            n214 = local read "Current Scale"() -> (w411:u16)
            n215 = in-place {
              in-place-border: w408 -> [w425]
              n216 = in-place-array #12(w414, w411) -> (w427:T3)
              n217 = Not Equal?(x=u16 5, y=w425) -> (x != y?=w423:bool)
              n218 = local write "Show Scale"(w423) -> ()
              n219 = Bundle By Name(cluster=w427, "General.Visible"=w423, "General.Style"=w425) -> (w426:T3)
              n220 = in-place-array #12(w426) -> (w413:T2)  [unwired: 1 out]
            }
            n221 = case shown="Default" w410 {
              tunnel: w412 -> [w417 _]
              tunnel: w411 -> [w416 _]
              tunnel: w409 -> [_ _]
              tunnel: w408 -> [w415 _]
              tunnel: [_ TRUE] -> w406
              frame Default {
                n222 = case shown="0, Default" w416 {
                  tunnel: w417 -> [w419 w421]
                  tunnel: w415 -> [w418 w420]
                  frame 0, Default {
                    n223 = property class="XYGraph (strict)"(reference=w419, "XScale.Style"=w418) -> ()  [unwired: 1 in, 2 out]
                  }
                  frame 1 {
                    n224 = property class="XYGraph (strict)"(reference=w421, "YScale.Style"=w420) -> ()  [unwired: 1 in, 2 out]
                  }
                }
              }
              frame 1 {
              }
            }
          }
          event "Major Tick", "Minor Tick": Value Change {
            n225 = event-data() -> ()  [unwired: 2 out]
            n226 = local read "Minor Tick"() -> (w429:u32)
            n227 = local read "Major Tick"() -> (w430:u32)
            n228 = local read "Current Scale"() -> (w433:u16)
            n229 = in-place {
              in-place-border: w430 -> [w451]
              in-place-border: w429 -> [w450]
              n230 = in-place-array #13(w436, w433) -> (w453:T3)
              n231 = Bundle By Name(cluster=w453, "Tick Color.Major Color"=w451, "Tick Color.Minor Color"=w450) -> (w452:T3)
              n232 = in-place-array #13(w452) -> (w435:T2)  [unwired: 1 out]
            }
            n233 = case shown="1" w432 {
              tunnel: w434 -> [w440 _]
              tunnel: w433 -> [w439 _]
              tunnel: w431 -> [_ w449]
              tunnel: w430 -> [w438 w448]
              tunnel: w429 -> [w437 w447]
              frame Default {
                n234 = case shown="1" w439 {
                  tunnel: w440 -> [w443 w445]
                  tunnel: w438 -> [w442 w446]
                  tunnel: w437 -> [w441 w444]
                  frame 0, Default {
                    n235 = property class="XYGraph (strict)"(reference=w443, "XScale.TickColor"=w442, "XScale.MinorTickColor"=w441) -> ()  [unwired: 1 in, 2 out]
                  }
                  frame 1 {
                    n236 = property class="XYGraph (strict)"(reference=w445, "YScale.TickColor"=w446, "YScale.MinorTickColor"=w444) -> ()  [unwired: 1 in, 2 out]
                  }
                }
              }
              frame 1 {
                n237 = property class="XYGraph (strict)"(reference=w449, "YScale.TickColor"=w448, "YScale.MinorTickColor"=w447) -> ()  [unwired: 1 in, 2 out]
              }
            }
          }
          event "Marker Text": Value Change {
            n238 = event-data() -> ("NewVal"=w455:u32)  [unwired: 1 out]
            n239 = local read "Current Scale"() -> (w458:u16)
            n240 = in-place {
              in-place-border: w455 -> [w471]
              n241 = in-place-array #14(w461, w458) -> (w473:T3)
              n242 = Bundle By Name(cluster=w473, "Marker.FG Color"=w471) -> (w472:T3)
              n243 = in-place-array #14(w472) -> (w460:T2)  [unwired: 1 out]
            }
            n244 = case shown="Default" w457 {
              tunnel: w459 -> [w464 _]
              tunnel: w458 -> [w463 _]
              tunnel: w456 -> [_ w470]
              tunnel: w455 -> [w462 w469]
              frame Default {
                n245 = case shown="1" w463 {
                  tunnel: w464 -> [w466 w468]
                  tunnel: w462 -> [w465 w467]
                  frame 0, Default {
                    n246 = property class="XYGraph (strict)"(reference=w466, "XScale.Text Color"=w465) -> ()  [unwired: 1 in, 2 out]
                  }
                  frame 1 {
                    n247 = property class="XYGraph (strict)"(reference=w468, "YScale.Text Color"=w467) -> ()  [unwired: 1 in, 2 out]
                  }
                }
              }
              frame 1 {
                n248 = property class="XYGraph (strict)"(reference=w470, "YScale.Text Color"=w469) -> ()  [unwired: 1 in, 2 out]
              }
            }
          }
          event "Grid Style": Value Change {
            n249 = event-data() -> ("NewVal"=w476:u16)  [unwired: 1 out]
            n250 = case shown="0" w476 {
              tunnel: w481 -> [w489 w509 w536]
              tunnel: [w488 w508 w535] -> w480
              tunnel: w479 -> [w487 w507 w534]
              tunnel: w478 -> [w485 w505 w532]
              tunnel: w477 -> [w484 w504 w531]
              tunnel: [w482 w501 w528] -> w474
              frame 0 {
                w483 = u32 16777216
                n251 = local read "Current Scale"() -> (w486:u16)
                n252 = local write "Major Grid"(w483) -> ()
                n253 = local write "Minor Grid"(w483) -> ()
                n254 = in-place {
                  in-place-border: w483 -> [w498]
                  n255 = in-place-array #15(w489, w486) -> (w500:T3)
                  n256 = Bundle By Name(cluster=w500, "Gird Color.Major Color"=w498, "Gird Color.Minor Color"=w498) -> (w499:T3)
                  n257 = in-place-array #15(w499) -> (w488:T2)  [unwired: 1 out]
                }
                n258 = case shown="Default" w485 {
                  tunnel: w487 -> [w492 _]
                  tunnel: w486 -> [w491 _]
                  tunnel: w484 -> [_ _]
                  tunnel: w483 -> [w490 _]
                  tunnel: [_ TRUE] -> w482
                  frame Default {
                    n259 = case shown="0, Default" w491 {
                      tunnel: w492 -> [w494 w496]
                      tunnel: w490 -> [w493 w495]
                      frame 0, Default {
                        n260 = property class="XYGraph (strict)"(reference=w494, "XScale.MajGrdColor"=w493, "XScale.MnrGrdColor"=w493) -> ()  [unwired: 1 in, 2 out]
                      }
                      frame 1 {
                        n261 = property class="XYGraph (strict)"(reference=w496, "YScale.MajGrdColor"=w495, "YScale.MnrGrdColor"=w495) -> ()  [unwired: 1 in, 2 out]
                      }
                    }
                  }
                  frame 1 {
                    # "Compass grids are drawn by image"
                  }
                }
              }
              frame 1 {
                w502 = u32 16777216
                n262 = local read "Current Scale"() -> (w506:u16)
                n263 = in-place {
                  in-place-border: w502 -> [w525]
                  in-place-border: [w521] -> w503
                  n264 = in-place-array #16(w509, w506) -> (w526:T3)
                  n265 = Unbundle By Name(w526) -> ("Gird Color.Major Color"=w522:u32)
                  n266 = Equal?(x=w525, y=w522) -> (x = y?=w524:bool)
                  n267 = Select(t=u32 9868950 ("Major Grid"), s=w524, f=w522) -> (s? t:f=w521:u32)
                  n268 = Bundle By Name(cluster=w526, "Gird Color.Minor Color"=w525, "Gird Color.Major Color"=w521) -> (w527:T3)
                  n269 = in-place-array #16(w527) -> (w508:T2)  [unwired: 1 out]
                }
                n270 = case shown="1" w505 {
                  tunnel: w507 -> [w513 _]
                  tunnel: w506 -> [w512 _]
                  tunnel: w504 -> [_ _]
                  tunnel: w502 -> [w511 _]
                  tunnel: w503 -> [w510 _]
                  tunnel: [_ TRUE] -> w501
                  frame Default {
                    n271 = case shown="0, Default" w512 {
                      tunnel: w513 -> [w516 w519]
                      tunnel: w511 -> [w515 w518]
                      tunnel: w510 -> [w514 w517]
                      frame 0, Default {
                        n272 = property class="XYGraph (strict)"(reference=w516, "XScale.MnrGrdColor"=w515, "XScale.MajGrdColor"=w514) -> ()  [unwired: 1 in, 2 out]
                      }
                      frame 1 {
                        n273 = property class="XYGraph (strict)"(reference=w519, "YScale.MnrGrdColor"=w518, "YScale.MajGrdColor"=w517) -> ()  [unwired: 1 in, 2 out]
                      }
                    }
                  }
                  frame 1 {
                    # "Compass grids are drawn by image"
                  }
                }
                n274 = local write "Major Grid"(w503) -> ()
                n275 = local write "Minor Grid"(w502) -> ()
              }
              frame 2, Default {
                n276 = local read "Current Scale"() -> (w533:u16)
                n277 = in-place {
                  in-place-border: [w553] -> w530
                  in-place-border: [w550] -> w529
                  w549 = u32 16777216
                  n278 = in-place-array #17(w536, w533) -> (w557:T3)
                  n279 = Unbundle By Name(w557) -> ("Gird Color.Major Color"=w554:u32, "Gird Color.Minor Color"=w548:u32)
                  n280 = Equal?(x=w549, y=w554) -> (x = y?=w556:bool)
                  n281 = Equal?(x=w549, y=w548) -> (x = y?=w552:bool)
                  n282 = Select(t=u32 9868950 ("Major Grid"), s=w556, f=w554) -> (s? t:f=w553:u32)
                  n283 = Select(t=u32 13816530 ("Minor Grid"), s=w552, f=w548) -> (s? t:f=w550:u32)
                  n284 = Bundle By Name(cluster=w557, "Gird Color.Major Color"=w553, "Gird Color.Minor Color"=w550) -> (w558:T3)
                  n285 = in-place-array #17(w558) -> (w535:T2)  [unwired: 1 out]
                }
                n286 = case shown="1" w532 {
                  tunnel: w534 -> [w540 _]
                  tunnel: w533 -> [w539 _]
                  tunnel: w531 -> [_ _]
                  tunnel: w529 -> [w538 _]
                  tunnel: w530 -> [w537 _]
                  tunnel: [_ TRUE] -> w528
                  frame Default {
                    n287 = case shown="0, Default" w539 {
                      tunnel: w540 -> [w543 w546]
                      tunnel: w538 -> [w542 w545]
                      tunnel: w537 -> [w541 w544]
                      frame 0, Default {
                        n288 = property class="XYGraph (strict)"(reference=w543, "XScale.MnrGrdColor"=w542, "XScale.MajGrdColor"=w541) -> ()  [unwired: 1 in, 2 out]
                      }
                      frame 1 {
                        n289 = property class="XYGraph (strict)"(reference=w546, "YScale.MnrGrdColor"=w545, "YScale.MajGrdColor"=w544) -> ()  [unwired: 1 in, 2 out]
                      }
                    }
                  }
                  frame 1 {
                    # "Compass grids are drawn by image"
                  }
                }
                n290 = local write "Major Grid"(w530) -> ()
                n291 = local write "Minor Grid"(w529) -> ()
              }
            }
          }
          event "Major Grid", "Minor Grid": Value Change {
            w567 = u32 16777216
            n292 = event-data() -> ()  [unwired: 2 out]
            n293 = local read "Major Grid"() -> (w566:u32)
            n294 = local read "Minor Grid"() -> (w565:u32)
            n295 = local read "Current Scale"() -> (w573:u16)
            n296 = Not Equal?(x=w566, y=w567) -> (x != y?=w569:bool)
            n297 = Not Equal?(x=w565, y=w567) -> (x != y?=w570:bool)
            n298 = in-place {
              in-place-border: w566 -> [w589]
              in-place-border: w565 -> [w588]
              n299 = in-place-array #18(w576, w573) -> (w591:T3)
              n300 = Bundle By Name(cluster=w591, "Gird Color.Major Color"=w589, "Gird Color.Minor Color"=w588) -> (w590:T3)
              n301 = in-place-array #18(w590) -> (w575:T2)  [unwired: 1 out]
            }
            n302 = case shown="Default" w572 {
              tunnel: w574 -> [w580 _]
              tunnel: w573 -> [w579 _]
              tunnel: w571 -> [_ _]
              tunnel: w566 -> [w578 _]
              tunnel: w565 -> [w577 _]
              tunnel: [_ TRUE] -> w559
              frame Default {
                n303 = case shown="1" w579 {
                  tunnel: w580 -> [w583 w585]
                  tunnel: w578 -> [w582 w586]
                  tunnel: w577 -> [w581 w584]
                  frame 0, Default {
                    n304 = property class="XYGraph (strict)"(reference=w583, "XScale.MajGrdColor"=w582, "XScale.MnrGrdColor"=w581) -> ()  [unwired: 1 in, 2 out]
                  }
                  frame 1 {
                    n305 = property class="XYGraph (strict)"(reference=w585, "YScale.MajGrdColor"=w586, "YScale.MnrGrdColor"=w584) -> ()  [unwired: 1 in, 2 out]
                  }
                }
              }
              frame 1 {
                # "Compass grids are drawn by image"
              }
            }
            n306 = Build Array(w569, w570) -> (w568:bool[])
            n307 = Boolean Array To Number(Boolean array=w568) -> (number=w561:u16)
            n308 = In Range and Coerce(upper limit=u16 2, x=w561, lower limit=u16 0) -> (coerced(x)=w560:u16)  [unwired: 1 out]
            n309 = local write "Grid Style"(w560) -> ()
          }
          event User Event {
            n310 = event-data() -> ()  [unwired: 2 out]
          }
        }
        n311 = case shown="True" w99 {
          tunnel: w101 -> [_ w108]
          frame False {
          }
          frame True {
            n312 = call <vilib>:"Temp Graph Update.vi"("Property Name"=Temp_Graph_Property_Action."Scales Property", "State"=Temp_Graph_State."Update Graph", "Property In"=w108) -> ()  [unwired: 2 in, 7 out]
          }
        }
      }
      frame "Exit" {
      }
    }
  }
  "Scale Array Out" <- w8
